vi "str to policy.vi"(2 "String":string) -> (6 "supported security policies (None)":T1={"None"=TRUE, "Sign with Basic128Rsa125"=FALSE, "Sign and Encrypt with Basic128Rsa125"=FALSE, "Sign with Basic256"=FALSE, "Sign and Encrypt with Basic256"=FALSE})   [LabVIEW 2013, in "CreateOPCUAServerAuto.lvlib"]
uses:
  CreateOPCUAServerAuto.lvlib
  <vilib>/OPCUA/server/subVI/supported security policies.ctl
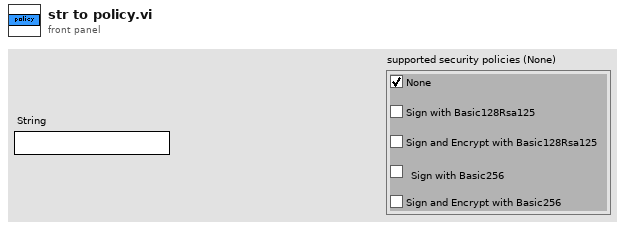
[diagram p1: front panel]
types:
  T1 = typedef "supported security policies.ctl" = cluster{"None":bool, "Sign with Basic128Rsa125":bool, "Sign and Encrypt with Basic128Rsa125":bool, "Sign with Basic256":bool, "Sign and Encrypt with Basic256":bool}
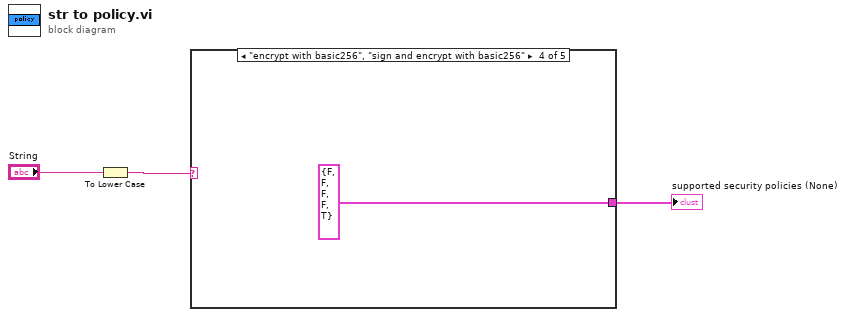
[diagram p0: block diagram]
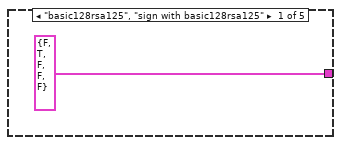
[diagram p2: hidden frame]
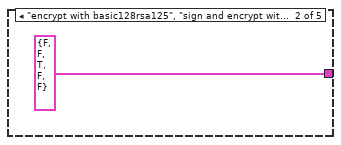
[diagram p3: hidden frame]
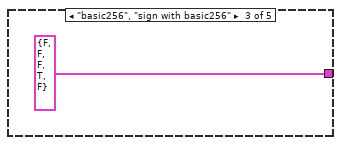
[diagram p4: hidden frame]
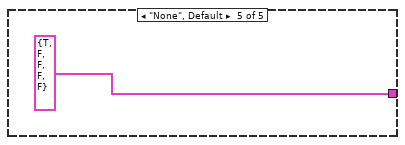
[diagram p5: hidden frame]
diagram:
  n1 = To Lower Case(string="String") -> (all lower case string=w1:string)
  n2 = case shown="\"encrypt with basic256\", \"sign and encrypt with basic256\"" w1 {
    tunnel: [T1 {"None"=FALSE, "Sign with Basic128Rsa125"=TRUE, "Sign and Encrypt with Basic128Rsa125"=FALSE, "Sign with Basic256"=FALSE, "Sign and Encrypt with Basic256"=FALSE} ("supported security policies (None)") T1 {"None"=FALSE, "Sign with Basic128Rsa125"=FALSE, "Sign and Encrypt with Basic128Rsa125"=TRUE, "Sign with Basic256"=FALSE, "Sign and Encrypt with Basic256"=FALSE} ("supported security policies (None)") T1 {"None"=FALSE, "Sign with Basic128Rsa125"=FALSE, "Sign and Encrypt with Basic128Rsa125"=FALSE, "Sign with Basic256"=TRUE, "Sign and Encrypt with Basic256"=FALSE} ("supported security policies (None)") T1 {"None"=FALSE, "Sign with Basic128Rsa125"=FALSE, "Sign and Encrypt with Basic128Rsa125"=FALSE, "Sign with Basic256"=FALSE, "Sign and Encrypt with Basic256"=TRUE} ("supported security policies (None)") T1 {"None"=TRUE, "Sign with Basic128Rsa125"=FALSE, "Sign and Encrypt with Basic128Rsa125"=FALSE, "Sign with Basic256"=FALSE, "Sign and Encrypt with Basic256"=FALSE} ("supported security policies (None)")] -> w3
    frame "basic128rsa125", "sign with basic128rsa125" {
    }
    frame "encrypt with basic128rsa125", "sign and encrypt with basic128rsa125" {
    }
    frame "basic256", "sign with basic256" {
    }
    frame "encrypt with basic256", "sign and encrypt with basic256" {
    }
    frame "None", Default {
    }
  }
  "supported security policies (None)" <- w3
